vi "Constructor.vi"(10 "Capacity 2^n":u32) -> (3 "POTTypedCircularBuffer out":refnum<class "POTTypedCircularBuffer.lvclass">)   [LabVIEW 2024, in "POTTypedCircularBuffer.lvclass"]
uses:
  POTTypedCircularBuffer.lvclass
  POTTypedCircularBuffer.lvclass/POTTypedCircularBuffer.ctl
  ReadCount.vi
  Reorder.vi
  ReadCapacity.vi
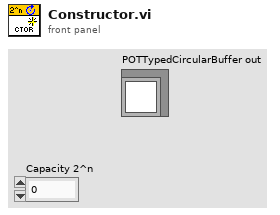
[diagram p1: front panel]
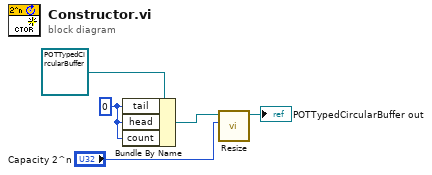
[diagram p0: block diagram]
diagram:
  w1 = 0 ("size")
  n1 = Bundle By Name(cluster=refnum<class "POTTypedCircularBuffer.lvclass"> refnum ("TypedCircularBuffer.lvclass"), "tail"=w1, "head"=w1, "count"=w1) -> (w4:refnum<class "POTTypedCircularBuffer.lvclass">)
  n2 = call "Resize.vi"("Capacity 2^n"="Capacity 2^n", "POTTypedCircularBuffer in"=w4) -> ("POTTypedCircularBuffer out"=→"POTTypedCircularBuffer out":refnum<class "POTTypedCircularBuffer.lvclass">)  [unwired: 9 in]
